vi "Shutter Core with Damping Option V2.vi"(4 "Shutter Drive":tag="Log/ao0", 5 "Thresholds":T1={"Legacy thrsh (nA)"=0.005, "Damped thrsh (nA)"=0.005} {"Damped thrsh (nA)" format="%.4f"; "Legacy thrsh (nA)" format="%.4f"}, 6 "Damping":bool=TRUE, 7 "Pulse Times":u16[][](array[numeric])=[[20, 70, 39, 54, 0, 100, 20], [20, 77, 33, 49, 0, 100, 20]], 8 "Legacy Pulse (ms)":u16=1000, 9 "Action":u16(ring) items=["Operate", "Initialize", "Read from .INI", "Write to .INI"], 10 "OPEN-CLOSE":bool, 11 "path to .INI file":path=path "D:/3D FIB-SEM Files/Jeiss.ini") -> (0 "error out":errorcluster, 1 "Legacy thrsh (nA)":dbl format="%.4f", 2 "Damped thrsh (nA)":dbl format="%.4f", 3 "file path Out":path)   [LabVIEW 2018]
uses:
  <vilib>/DAQmx/write.llb/DAQmx Write (Analog 1D DBL 1Chan NSamp).vi
  <vilib>/DAQmx/create/channels.llb/DAQmx Create Channel (AO-Voltage-Basic).vi
  <vilib>/DAQmx/configure/timing.llb/DAQmx Timing (Sample Clock).vi
  <vilib>/DAQmx/miscellaneous.llb/DAQmx Fill In Error Info.vi
panel:
  out "Waveform Graph":dbl[](graph)
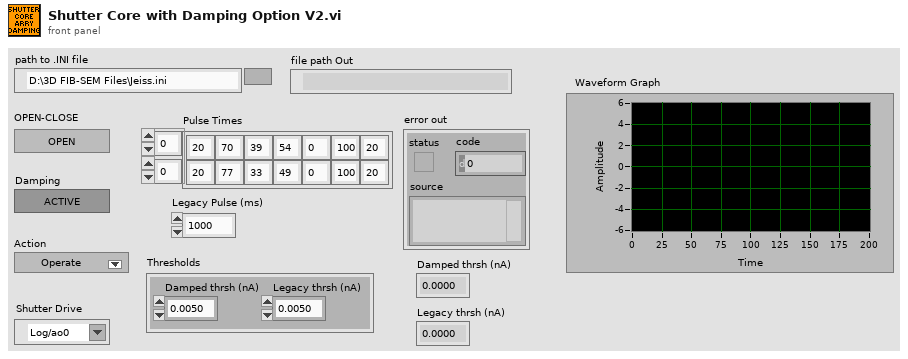
[diagram p1: front panel]
types:
  T1 = cluster{"Legacy thrsh (nA)":dbl, "Damped thrsh (nA)":dbl}
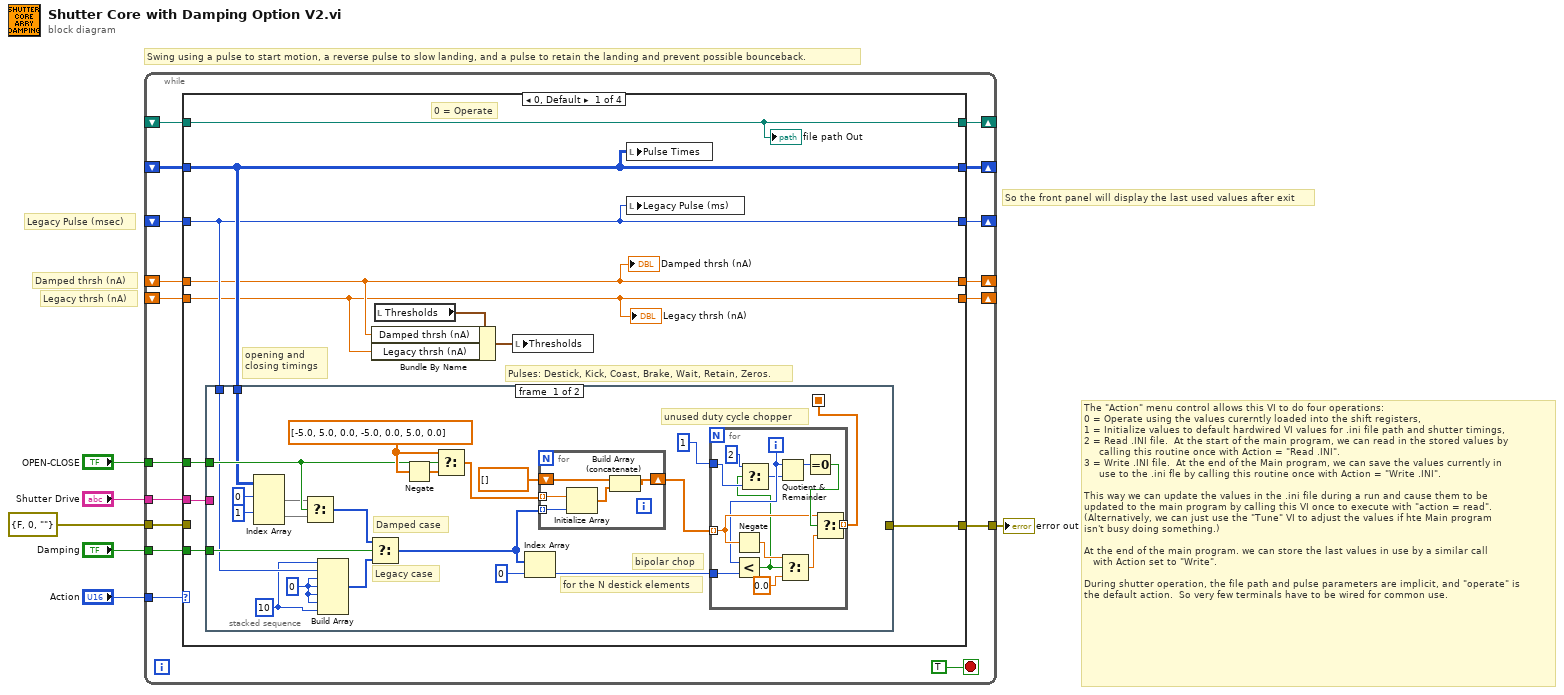
[diagram p0: block diagram]
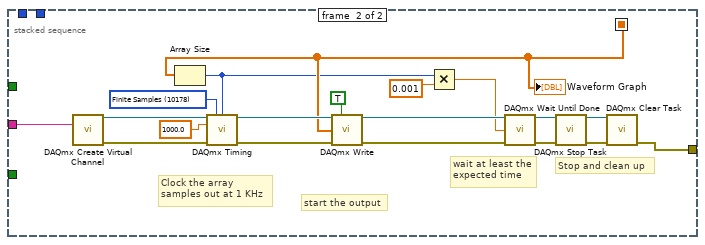
[diagram p2: hidden frame]
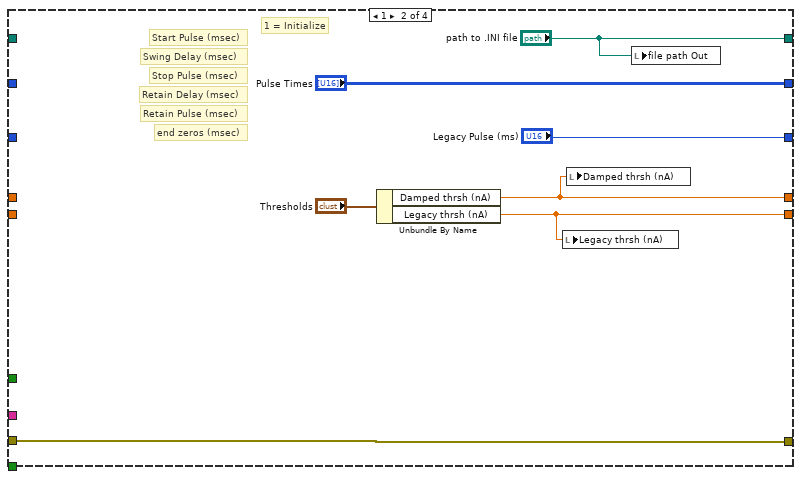
[diagram p3: hidden frame]
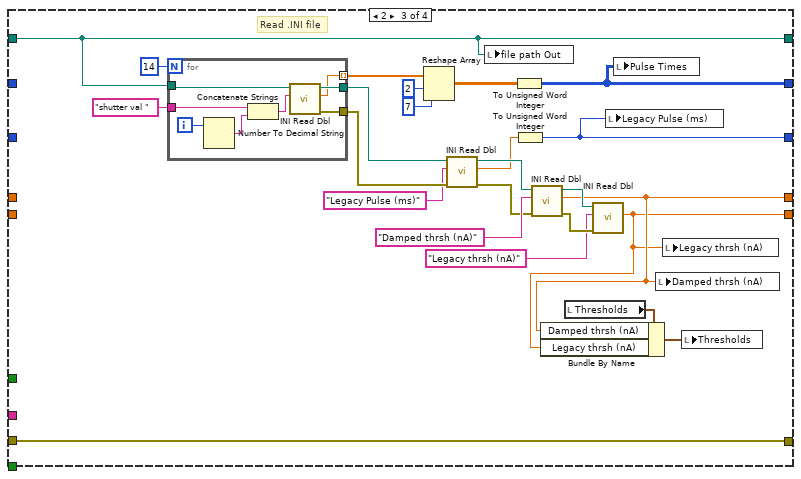
[diagram p4: hidden frame]
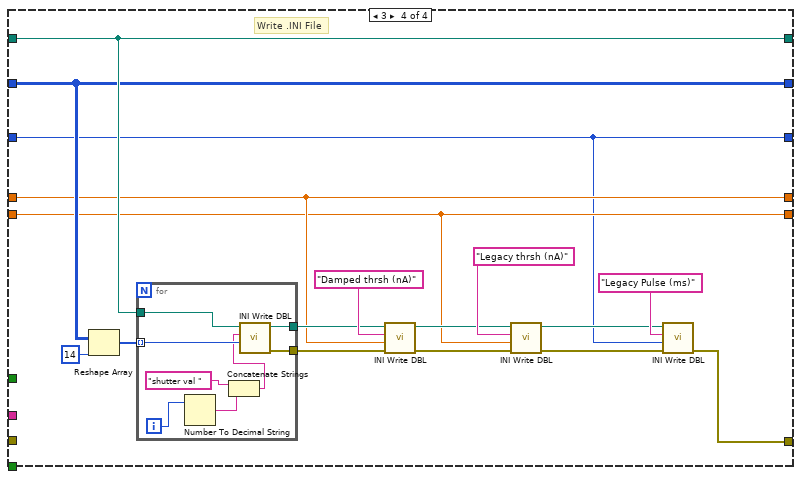
[diagram p5: hidden frame]
diagram:
  # "Legacy Pulse (msec)"
  # "Legacy thrsh (nA)"
  # "Damped thrsh (nA)"
  # "So the front panel will display the last used values after exit"
  # "Swing using a pulse to start motion, a reverse pulse to slow landing, and a pulse to retain the landing and prevent possible bounceback."
  # "The \"Action\" menu control allows this VI to do four operations:\n0 = Operate using the values curerntly loaded into the shift registers,\n1 = Initialize values to default hardwired VI values for .ini file path and shutter timings,\n2 = Read .INI file.  At the start of the main program, we can read in the stored values by\n     calling this routine once with Action = \"Read .INI\".\n3 = Write .INI file.  At the end of the Main program, we can save the values currently in\n     use to the .ini fle by calling this routine once with Action = \"Write .INI\".\n\nThis way we can update the values in the .ini file during a run and cause them to be \nupdated to the main program by calling this VI once to execute with \"action = read\".\n(Alternatively, we can just use the \"Tune\" VI to adjust the values if hte Main program\nisn't busy doing something.)\n\nAt the end of the main program. we can store the last values in use by a similar call\n   with Action set to \"Write\".\n\nDuring shutter operation, the file path and pulse parameters are implicit, and \"operate\" is \nthe default action.  So very few terminals have to be wired for common use."
  n1 = while {
    tunnel: "Damping" -> [w23]
    tunnel: errorcluster {"status"=FALSE, "code"=0, "source"=""} ("error in") -> [w22]
    tunnel: "OPEN-CLOSE" -> [w21]
    shift-right: [w19] -> _
    shift-left: _ -> [w18]
    tunnel: "Action" -> [w20]
    tunnel: [w17] -> w3
    shift-right: [w15] -> _
    shift-left: _ -> [w16]
    tunnel: "Shutter Drive" -> [w14]
    shift-right: [w12] -> _
    shift-left: _ -> [w13]
    shift-right: [w10] -> _
    shift-left: _ -> [w11]
    shift-right: [w8] -> _
    shift-left: _ -> [w7]
    stop <- TRUE stop-if-true
    n2 = case shown="0, Default" w20 {
      tunnel: w23 -> [w33 _ _ _]
      tunnel: w22 -> [_ w100 w108 _]
      tunnel: w21 -> [w34 _ _ _]
      tunnel: [w30 "Pulse Times" w105 w136] -> w19
      tunnel: w18 -> [w30 _ _ w136]
      tunnel: [w29 "Legacy Pulse (ms)" w104 w133] -> w8
      tunnel: w7 -> [w29 _ _ w133]
      tunnel: [w31 w100 w108 w138] -> w17
      tunnel: w16 -> [w24 _ w101 w137]
      tunnel: [w24 "path to .INI file" w101 w137] -> w15
      tunnel: w14 -> [w32 _ _ _]
      tunnel: w13 -> [w26 _ _ w135]
      tunnel: [w26 w95 w103 w135] -> w12
      tunnel: w11 -> [w25 _ _ w134]
      tunnel: [w25 w96 w102 w134] -> w10
      frame 0, Default {
        # "Pulses: Destick, Kick, Coast, Brake, Wait, Retain, Zeros."
        # "opening and\nclosing timings"
        # "0 = Operate"
        n3 = stacked-sequence {
          seq-local: [w43 _] -> [_ w77]
          tunnel: w34 -> [w51 _]
          tunnel: w30 -> [w50 _]
          tunnel: w33 -> [w55 _]
          tunnel: w32 -> [_ w80]
          tunnel: [_ w79] -> w31
          tunnel: w29 -> [w42 _]
          frame #0 {
            w41 = u16 0 ("element")
            w36 = u16 10 ("element")
            w52 = dbl[] [-5.0, 5.0, 0.0, -5.0, 0.0, 5.0, 0.0]
            # "bipolar chop"
            # "for the N destick elements"
            # "unused duty cycle chopper"
            # "Damped case"
            # "Legacy case"
            n4 = Index Array(array=w50, index (row) #1=0 ("index (row)"), index (row) #2=1 ("index (row)")) -> (element #1=w49:u16[], element #2=w48:u16[])  [unwired: 2 in]
            n5 = Select(t=w49, s=w51, f=w48) -> (s? t:f=w45:u16[])
            n6 = Build Array(w36, w42, w41, w41, w41, w41, w36) -> (w54:u16[])
            n7 = Select(t=w45, s=w55, f=w54) -> (s? t:f=w40:u16[])
            n8 = Negate(x=w52) -> (-x=w53:dbl[])
            n9 = Select(t=w52, s=w51, f=w53) -> (s? t:f=w37:dbl[])
            n10 = Index Array(array=w40, index=0) -> (element=w38:u16)
            n11 = for {
              tunnel: w37 -> [w71] mode=indexing
              tunnel: w40 -> [w74] mode=indexing
              shift-right: [w73] -> w44
              shift-left: dbl[] [] -> [w72]
              n12 = Initialize Array(w71, w74) -> (w70:dbl[])
              n13 = Build Array (concatenate)(w72, w70) -> (w73:dbl[])
            }
            n14 = for {
              tunnel: w44 -> [w63] mode=indexing
              tunnel: u8 1 ("t") -> [w60]
              tunnel: [w67] -> w43 mode=indexing
              tunnel: w38 -> [w66]
              i -> [w61]
              n15 = Negate(x=w63) -> (-x=w62:dbl)
              n16 = Less?(x=w61, y=w66) -> (x < y?=w58:bool)
              n17 = Select(t=u8 2, s=w58, f=w60) -> (s? t:f=w59:u8)
              n18 = Quotient & Remainder(x=w61, y=w59) -> (x-y*floor(x/y)=w69:i32)  [unwired: 1 out]
              n19 = Select(t=w62, s=w58, f=0.0) -> (s? t:f=w64:dbl)
              n20 = Equal To 0?(x=w69) -> (x = 0?=w68:bool)
              n21 = Select(t=w63, s=w68, f=w64) -> (s? t:f=w67:dbl)
            }
          }
          frame #1 {
            w85 = 10178 items=["Finite Samples"=10178, "Continuous Samples"=10123, "Hardware Timed Single Point"=12522] ("sample mode")
            # "Stop and clean up"
            # "wait at least the\nexpected time"
            # "start the output"
            # "Clock the array \nsamples out at 1 KHz"
            n22 = call-poly <vilib>:"DAQmx Create Virtual Channel.vi"("physical channels"=w80) -> ("task out"=w83:refnum<k21>, "error out"=w84:errorcluster)  [unwired: 13 in]
            n23 = Array Size(array=w77) -> (size(s)=w75:i32)
            n24 = call-poly <vilib>:"DAQmx Timing.vi"("task/channels in"=w83, "sample mode"=w85, "samples per channel"=w75, "rate"=1000.0, "error in"=w84) -> ("task out"=w86:refnum<k21>, "error out"=w87:errorcluster)  [unwired: 9 in]
            n25 = call-poly <vilib>:"DAQmx Write.vi"("task/channels in"=w86, "auto start"=TRUE, "data"=w77, "error in"=w87) -> ("task out"=w90:refnum<k21>, "error out"=w91:errorcluster)  [unwired: 9 in, 1 out]
            n26 = Multiply(x=w75, y=0.001 ("timeout (sec)")) -> (x*y=w78:dbl)
            n27 = call <vilib>:"DAQmx Wait Until Done.vi"("task/channels in"=w90, "timeout (sec)"=w78, "error in"=w91) -> ("task out"=w93:refnum<k21>, "error out"=w92:errorcluster)  [unwired: 11 in]
            n28 = call <vilib>:"DAQmx Stop Task.vi"("task/channels in"=w93, "error in"=w92) -> ("task out"=w81:refnum<k21>, "error out"=w82:errorcluster)  [unwired: 12 in]
            n29 = call <vilib>:"DAQmx Clear Task.vi"("task in"=w81, "error in"=w82) -> ("error out"=w79:errorcluster)  [unwired: 13 in]
            "Waveform Graph" <- w77
          }
        }
        n30 = local read "Thresholds"() -> (w27:T1)
        n31 = Bundle By Name(cluster=w27, "Damped thrsh (nA)"=w26, "Legacy thrsh (nA)"=w25) -> (w28:T1)
        n32 = local write "Thresholds"(w28) -> ()
        n33 = local write "Pulse Times"(w30) -> ()
        n34 = local write "Legacy Pulse (ms)"(w29) -> ()
        "Damped thrsh (nA)" <- w26
        "Legacy thrsh (nA)" <- w25
        "file path Out" <- w24
      }
      frame 1 {
        # "end zeros (msec)"
        # "Retain Pulse (msec)"
        # "Retain Delay (msec)"
        # "Stop Pulse (msec)"
        # "Swing Delay (msec)"
        # "Start Pulse (msec)"
        # "1 = Initialize"
        n35 = Unbundle By Name("Thresholds") -> ("Damped thrsh (nA)"=w95:dbl, "Legacy thrsh (nA)"=w96:dbl)
        n36 = local write "Legacy thrsh (nA)"(w96) -> ()
        n37 = local write "Damped thrsh (nA)"(w95) -> ()
        n38 = local write "file path Out"("path to .INI file") -> ()
      }
      frame 2 {
        # "Read .INI file"
        n39 = for {
          N: 14 -> [_]
          tunnel: w101 -> [w129]
          tunnel: "shutter val " ("Key Str") -> [w128]
          tunnel: [w127] -> w123
          tunnel: [w126] -> w114 mode=indexing
          tunnel: [w125] -> w124
          i -> [w132]
          n40 = Number To Decimal String(number=w132) -> (decimal integer string=w131:string)  [unwired: 1 in]
          n41 = Concatenate Strings(w128, w131) -> (w130:string)
          n42 = call "INI Read Dbl.vi"("Key Str"=w130, "configuration file path"=w129) -> ("error out"=w125:errorcluster, "Value Out"=w126:dbl, "file path Out"=w127:path)  [unwired: 7 in]
        }
        n43 = Reshape Array(w114, 2 ("dimension size"), 7 ("dimension size")) -> (w111:dbl[][])
        n44 = call "INI Read Dbl.vi"("error IN"=w124, "Key Str"="Legacy Pulse (ms)", "configuration file path"=w123) -> ("error out"=w117:errorcluster, "Value Out"=w109:dbl, "file path Out"=w119:path)  [unwired: 6 in]
        n45 = local write "file path Out"(w101) -> ()
        n46 = To Unsigned Word Integer(number=w111) -> (unsigned 16bit integer=w105:u16[][])
        n47 = To Unsigned Word Integer(number=w109) -> (unsigned 16bit integer=w104:u16)
        n48 = call "INI Read Dbl.vi"("error IN"=w117, "Key Str"="Damped thrsh (nA)", "configuration file path"=w119) -> ("error out"=w118:errorcluster, "Value Out"=w103:dbl, "file path Out"=w120:path)  [unwired: 6 in]
        n49 = local read "Thresholds"() -> (w106:T1)
        n50 = call "INI Read Dbl.vi"("error IN"=w118, "Key Str"="Legacy thrsh (nA)", "configuration file path"=w120) -> ("Value Out"=w102:dbl)  [unwired: 6 in, 2 out]
        n51 = Bundle By Name(cluster=w106, "Damped thrsh (nA)"=w103, "Legacy thrsh (nA)"=w102) -> (w107:T1)
        n52 = local write "Legacy Pulse (ms)"(w104) -> ()
        n53 = local write "Pulse Times"(w105) -> ()
        n54 = local write "Damped thrsh (nA)"(w103) -> ()
        n55 = local write "Legacy thrsh (nA)"(w102) -> ()
        n56 = local write "Thresholds"(w107) -> ()
      }
      frame 3 {
        # "Write .INI File"
        n57 = Reshape Array(w136, 14 ("dimension size")) -> (w140:u16[])
        n58 = for {
          tunnel: w140 -> [w157] mode=indexing
          tunnel: [w152] -> w141
          tunnel: [w151] -> w145
          tunnel: w137 -> [w150]
          i -> [w156]
          n59 = Number To Decimal String(number=w156) -> (decimal integer string=w155:string)  [unwired: 1 in]
          n60 = Concatenate Strings("shutter val " ("Key Str"), w155) -> (w153:string)
          n61 = call "INI Write DBL.vi"("Value In"=w157, "Key Str"=w153, "configuration file path"=w150) -> ("error out"=w151:errorcluster, "file path Out"=w152:path)  [unwired: 7 in]
        }
        n62 = call "INI Write DBL.vi"("error IN"=w145, "Value In"=w135, "Key Str"="Damped thrsh (nA)", "configuration file path"=w141) -> ("error out"=w146:errorcluster, "file path Out"=w143:path)  [unwired: 6 in]
        n63 = call "INI Write DBL.vi"("error IN"=w146, "Value In"=w134, "Key Str"="Legacy thrsh (nA)", "configuration file path"=w143) -> ("error out"=w148:errorcluster, "file path Out"=w147:path)  [unwired: 6 in]
        n64 = call "INI Write DBL.vi"("error IN"=w148, "Value In"=w133, "Key Str"="Legacy Pulse (ms)", "configuration file path"=w147) -> ("error out"=w138:errorcluster)  [unwired: 6 in, 1 out]
      }
    }
  }
  "error out" <- w3
